vi "Create Client.vi"(8 "error in (no error)":errorcluster, 9 "TCP":refnum<k5>, 10 "Request":refnum<class "Request.lvclass">, 11 "WebSocket Manager in":refnum<class "WebSocket Manager.lvclass">) -> (0 "error out":errorcluster, 2 "WS Client":refnum<class "WebSocket Client.lvclass">)   [LabVIEW 2020, in "HTTP Server.lvlib" / "WebSocket Manager.lvclass"]
uses:
  WebSocket Manager.lvclass
  lv-http-util/HTTP Utils/Request/Request.lvclass
  WebSocket Client/WebSocket Client.lvclass
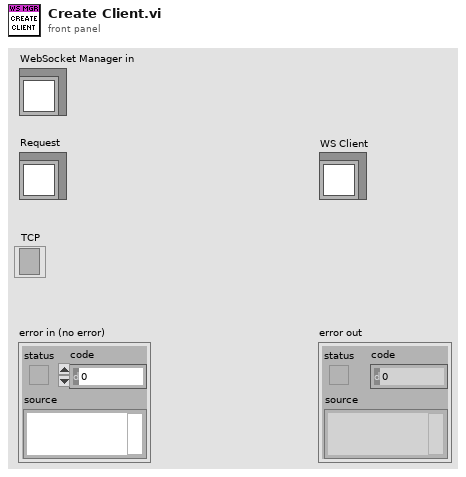
[diagram p1: front panel]
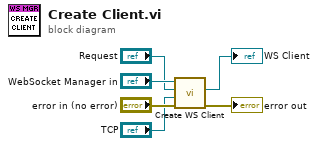
[diagram p0: block diagram]
diagram:
  n1 = call-dynamic "Create WS Client.vi"("error in (no error)"="error in (no error)", "TCP"="TCP", "Request"="Request", "WebSocket Manager in"="WebSocket Manager in") -> ("error out"=→"error out":errorcluster, "WS Client"=→"WS Client":refnum<class "WebSocket Client.lvclass">)  [unwired: 6 in]
